vi "Gaussian Blur.vi"(9 "Standard Deviation":dbl=1.0, 10 "Kernel Size":i32=11, 11 "Image":T1) -> (3 "Image Out":T1)   [LabVIEW 2011]
uses:
  <vilib>/vision/Image Controls.llb/IMAQ Image.ctl
  <vilib>/Analysis/2dsp.llb/2D Convolution (DBL).vi
  <vilib>/Analysis/NI_AALPro.lvlib
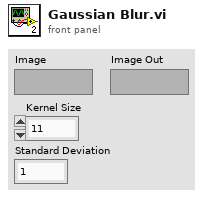
[diagram p1: front panel]
types:
  T1 = typedef "IMAQ Image.ctl" = refnum<image>
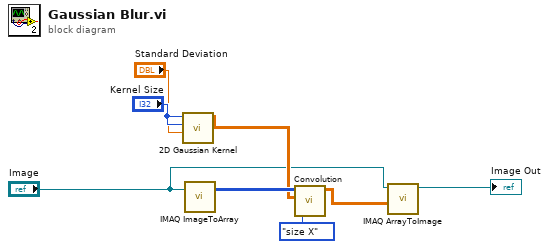
[diagram p0: block diagram]
diagram:
  n1 = call "2D Gaussian Kernel.vi"("Standard Deviation"="Standard Deviation", "Gaussian Kernel Y Dimension"="Kernel Size", "Gaussian Kernel X Dimension"="Kernel Size") -> ("Kernel"=w5:dbl[][])  [unwired: 8 in]
  n2 = call "IMAQ ImageToArray"("Image"="Image") -> ("Image Pixels (I16)"=w6:i16[][])  [unwired: 3 in, 4 out]
  n3 = call-poly <vilib>:"Convolution.vi"("output size"=enum32{"full", "size X", "compact"}."size X", "Y"=w5, "X"=w6) -> ("X * Y"=w3:dbl[][])  [unwired: 7 in, 1 out]
  n4 = call "IMAQ ArrayToImage"("Image Pixels (I16)"=w3, "Image"="Image") -> ("Image Out"=→"Image Out":T1)  [unwired: 8 in, 1 out]
